vi "MGCC_StaEst_funDSE_sub1.vi"(0 "MeaEqu":dbl[](array[numeric]), 3 "Weight":dbl[][](array[numeric]), 4 "measure":dbl[](array[numeric]), 5 "Num":T1, 6 "equ_vn":dbl[](array[numeric]), 7 "equ_qn":dbl[](array[numeric]), 8 "equ_pn":dbl[](array[numeric]), 9 "joc_vn":dbl[][](array[numeric]), 10 "joc_qn":dbl[][](array[numeric]), 11 "joc_pn":dbl[][](array[numeric])) -> (1 "G3":dbl[][](array[numeric]), 2 "G2":dbl[](array[numeric]))   [LabVIEW 2016]
uses:
  <vilib>/Analysis/baseanly.llb/A x Vector.vi
  <vilib>/imath/engines/lvmath2/RunTimeEngine/RunTimeType/NIMS_RunTimeType_From StrictType (excl LVString).vi
  <instcachedir>/0/NIMS_RunTimeType_From StrictType (excl LVString)_BBF44FB49F834B71AF7A14CCEDF8BECD.lvgen/NIMS_RunTimeType_From StrictType (excl LVString)_BBF44FB49F834B71AF7A14CCEDF8BECD_032.vi
  <instcachedir>/0/NIMS_RunTimeType_From StrictType (excl LVString)_BBF44FB49F834B71AF7A14CCEDF8BECD.lvgen/NIMS_RunTimeType_From StrictType (excl LVString)_BBF44FB49F834B71AF7A14CCEDF8BECD_031.vi
  <vilib>/imath/engines/lvmath2/RunTimeEngine/Struct/NIMS_StructSetField.vi
  <vilib>/imath/engines/lvmath2/RunTimeEngine/Struct/NIMS_StructGetField.vi
  <vilib>/imath/engines/lvmath2/RunTimeEngine/RunTimeType/NIMS_RunTimeType_To Numeric.vi
  <instcachedir>/0/NIMS_RunTimeType_To Numeric_19D51BCABB82435A94073491761E42EE.lvgen/NIMS_RunTimeType_To Numeric_19D51BCABB82435A94073491761E42EE_009.vi
  <instcachedir>/0/NIMS_RunTimeType_To Numeric_19D51BCABB82435A94073491761E42EE.lvgen/NIMS_RunTimeType_To Numeric_19D51BCABB82435A94073491761E42EE_008.vi
  <vilib>/imath/engines/lvmath2/RunTimeEngine/MatrixToken/NIMS_MatrixToken_M_M.vi
  <instcachedir>/0/NIMS_MatrixToken_M_M_DF273B0CC20F424BBF1EDA9F4E71C841.lvgen/NIMS_MatrixToken_M_M_DF273B0CC20F424BBF1EDA9F4E71C841_004.vi
  <vilib>/imath/engines/lvmath2/RunTimeEngine/ErrorHandling/NIMS_Create Error From Enums.vi
  <vilib>/imath/engines/lvmath2/RunTimeEngine/RangeToken/NIMS_Range.vi
  <instcachedir>/0/NIMS_Range_A7C094595B484CA7AF10685B02D808ED.lvgen/NIMS_Range_A7C094595B484CA7AF10685B02D808ED_000.vi
  <vilib>/imath/engines/lvmath2/RunTimeEngine/IndexReplace/NIMS M($,V)=S.vi
  <instcachedir>/0/NIMS M($,V)=S_8FF4B0FF94A24B3598424F2A899DBD06.lvgen/NIMS M($,V)=S_8FF4B0FF94A24B3598424F2A899DBD06_000.vi
  <vilib>/imath/engines/lvmath2/RunTimeSupport/NIMS_Error if Not Equal.vi
  <instcachedir>/0/NIMS_Error if Not Equal_43252A79AD05436189442EC0C5E5AB8A.lvgen/NIMS_Error if Not Equal_43252A79AD05436189442EC0C5E5AB8A_001.vi
  <vilib>/imath/engines/lvmath2/RunTimeEngine/ArithmeticOperatorToken/NIMS_ArithmeticOperator_minus.vi
  <instcachedir>/0/NIMS_ArithmeticOperator_minus_E3B65B1D26A44BB184AFDC5B3F458E3D.lvgen/NIMS_ArithmeticOperator_minus_E3B65B1D26A44BB184AFDC5B3F458E3D_003.vi
  <vilib>/imathl/engines/lvmath/Functions/Error Handling/Create Error.vi
  <vilib>/imath/engines/lvmath2/RunTimeEngine/NodeEndStatement/NIMS_NodeEndStatement_Output.vi
  <instcachedir>/0/NIMS_NodeEndStatement_Output_53EC0D466D134D7ABD903AC30B43404B.lvgen/NIMS_NodeEndStatement_Output_53EC0D466D134D7ABD903AC30B43404B_005.vi
  <instcachedir>/0/NIMS_NodeEndStatement_Output_53EC0D466D134D7ABD903AC30B43404B.lvgen/NIMS_NodeEndStatement_Output_53EC0D466D134D7ABD903AC30B43404B_002.vi
  <instcachedir>/0/NIMS_NodeEndStatement_Output_53EC0D466D134D7ABD903AC30B43404B.lvgen/NIMS_NodeEndStatement_Output_53EC0D466D134D7ABD903AC30B43404B_011.vi
  <instcachedir>/0/NIMS_NodeEndStatement_Output_53EC0D466D134D7ABD903AC30B43404B.lvgen/NIMS_NodeEndStatement_Output_53EC0D466D134D7ABD903AC30B43404B_018.vi
  <vilib>/imath/engines/lvmath2/RunTimeEngine/ErrorHandling/NIMS_Finalize Error.vi
  <vilib>/imath/engines/lvmath2/RunTimeEngine/ArithmeticOperatorToken/NIMS_ArithmeticOperator_rightdivmx.vi
  <instcachedir>/0/NIMS_ArithmeticOperator_rightdivmx_0DBBD6F2821B4AB59571CD9AB2DE9D62.lvgen/NIMS_ArithmeticOperator_rightdivmx_0DBBD6F2821B4AB59571CD9AB2DE9D62_000.vi
  <vilib>/imath/engines/lvmath2/RunTimeEngine/ArithmeticOperatorToken/NIMS_ArithmeticOperator_multmx.vi
  <instcachedir>/0/NIMS_ArithmeticOperator_multmx_4A56FE5C615140CE835D4DB5891BF065.lvgen/NIMS_ArithmeticOperator_multmx_4A56FE5C615140CE835D4DB5891BF065_004.vi
  <vilib>/Analysis/NI_AALBase.lvlib
panel:
  out "De size(s)":i32
  out "W size(s)":i32[](array[numeric])
  out "H size(s)":i32[](array[numeric])
  out "H":dbl[][](array[numeric])
  out "error out 2":errorcluster
  out "error out":errorcluster
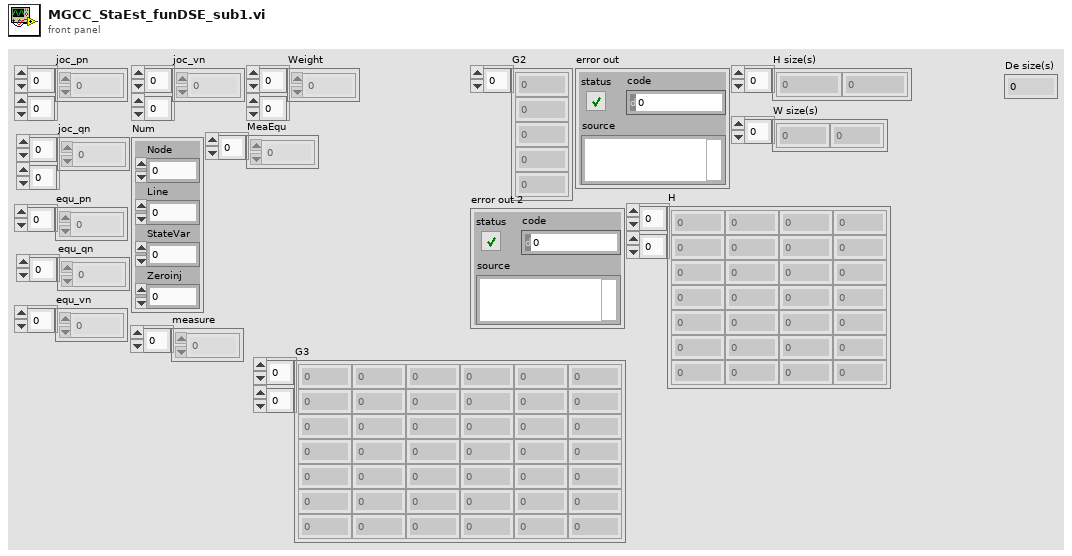
[diagram p1: front panel]
types:
  T1 = cluster{"Node":dbl, "Line":dbl, "StateVar":i32, "Zeroinj":i32}
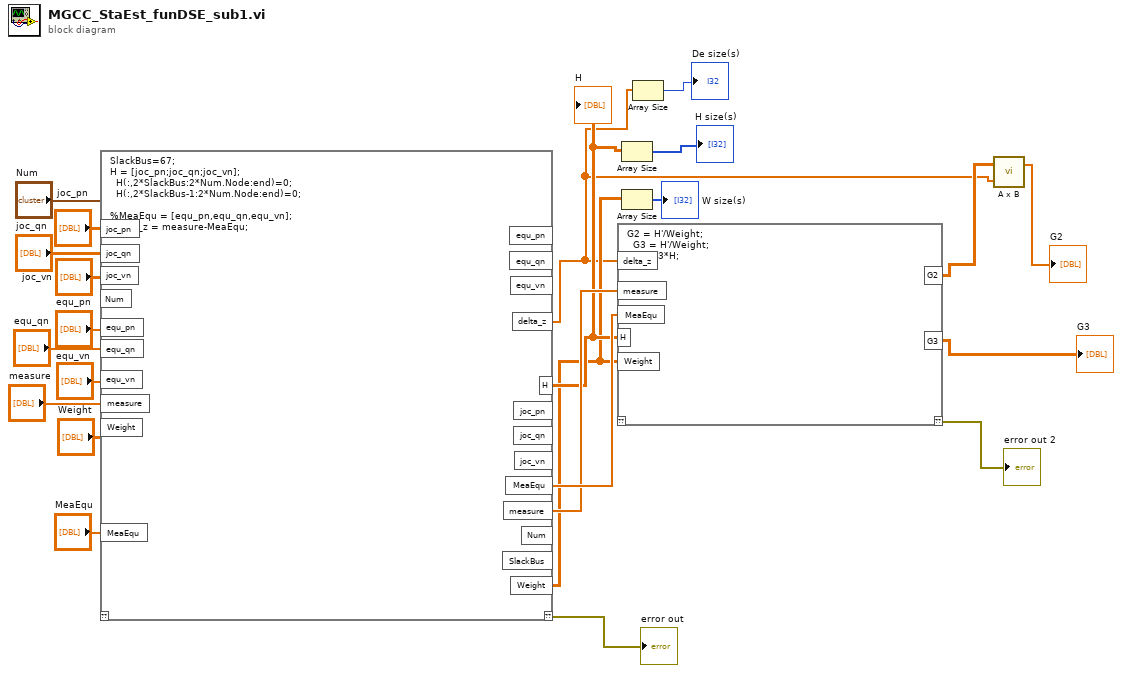
[diagram p0: block diagram]
diagram:
  n1 = mathscript code="SlackBus=67;  \nH = [joc_pn;joc_qn;joc_vn];\n  H(:,2*SlackBus:2*Num.Node:end)=0;   \n  H(:,2*SlackBus-1:2*Num.Node:end)=0; \n\n%MeaEqu = [equ_pn,equ_qn,equ_vn];\n delta_z = measure-MeaEqu;"("joc_pn"="joc_pn", "joc_qn"="joc_qn", "joc_vn"="joc_vn", "Num"="Num", "equ_pn"="equ_pn", "equ_qn"="equ_qn", "equ_vn"="equ_vn", "measure"="measure", "Weight"="Weight", "MeaEqu"="MeaEqu") -> ("??"=→"error out":errorcluster, "H"=w8:dbl[][], "MeaEqu"=w12:dbl[], "measure"=w11:dbl[], "Weight"=w6:dbl[][], "delta_z"=w2:dbl[])  [unwired: 1 in, 8 out]
  "H" <- w8
  n2 = mathscript code="G2 = H'/Weight;\n  G3 = H'/Weight;\n G3=G3*H;"("measure"=w11, "MeaEqu"=w12, "H"=w8, "Weight"=w6, "delta_z"=w2) -> ("??"=→"error out 2":errorcluster, "G2"=w3:dbl[][], "G3"=→"G3":dbl[][])  [unwired: 1 in]
  n3 = Array Size(array=w8) -> (size(s)=→"H size(s)":i32[])
  n4 = Array Size(array=w6) -> (size(s)=→"W size(s)":i32[])
  n5 = Array Size(array=w2) -> (size(s)=→"De size(s)":i32)
  n6 = call-poly <vilib>:"A x B.vi"("Vector"=w2, "A"=w3) -> ("A x Vector"=→"G2":dbl[])  [unwired: 1 out]
